vi "Rotate_3D_object.vi"(8 "error in (no error)":errorcluster, 10 "Orientation (pitch, roll, yaw)":dbl[](array[numeric]), 11 "SceneObject in":refnum<vi>) -> (0 "error out":errorcluster, 3 "SceneObject out":refnum<vi>)   [LabVIEW 2014]
uses:
  <vilib>/picture/3D Picture Control/NI_3D Picture Control.lvlib
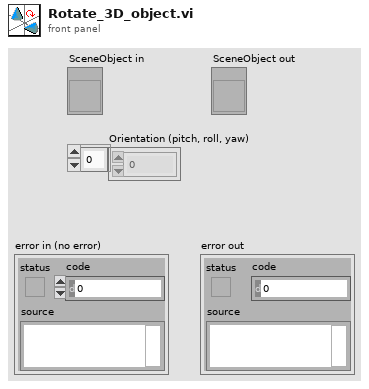
[diagram p1: front panel]
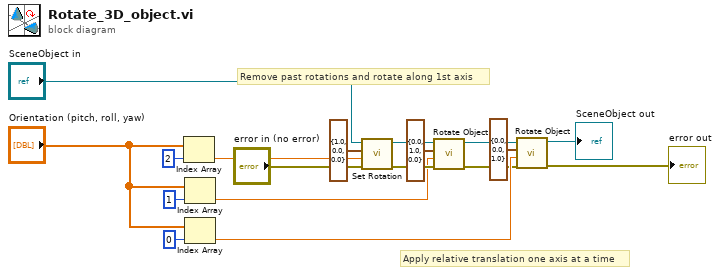
[diagram p0: block diagram]
diagram:
  # "Remove past rotations and rotate along 1st axis"
  # "Apply relative translation one axis at a time"
  n1 = Index Array(array="Orientation (pitch, roll, yaw)", index=2) -> (element=w6:dbl)
  n2 = Index Array(array="Orientation (pitch, roll, yaw)", index=1) -> (element=w1:dbl)
  n3 = Index Array(array="Orientation (pitch, roll, yaw)", index=0) -> (element=w17:dbl)
  n4 = call <vilib>:"Set Rotation.vi"("error in (no error)"="error in (no error)", "Angle"=w6, "Axis"=cluster{"X":sgl, "Y":sgl, "Z":sgl} {"X"=1.0, "Y"=0.0, "Z"=0.0}, "Scene Object"="SceneObject in") -> ("error out"=w3:errorcluster, "Rotated Scene Object"=w4:refnum<vi>)  [unwired: 6 in]
  n5 = call <vilib>:"Rotate Object.vi"("error in (no error)"=w3, "Angle"=w1, "Axis"=cluster{"X":sgl, "Y":sgl, "Z":sgl} {"X"=0.0, "Y"=1.0, "Z"=0.0}, "Scene.Object In"=w4) -> ("error out"=w10:errorcluster, "Scene.Object Out"=w16:refnum<vi>)  [unwired: 6 in]
  n6 = call <vilib>:"Rotate Object.vi"("error in (no error)"=w10, "Angle"=w17, "Axis"=cluster{"X":sgl, "Y":sgl, "Z":sgl} {"X"=0.0, "Y"=0.0, "Z"=1.0}, "Scene.Object In"=w16) -> ("error out"=→"error out":errorcluster, "Scene.Object Out"=→"SceneObject out":refnum<vi>)  [unwired: 6 in]
